vi "Release Buffer.vi"(8 "error in (no error)":errorcluster, 11 "buffer":refnum<data-value>) -> (0 "error out":errorcluster)   [LabVIEW 2017, in "Waveforms (N Ch).lvclass"]
doc: "Releases a reference to a buffer of continuous waveforms. Use this VI to clear all data from the buffer and destroy the buffer reference."
uses:
  <vilib>/addons/_NISVFA/_Shared subVIs/Data Objects/Waveforms (DBL)/Waveforms (N Ch).lvclass
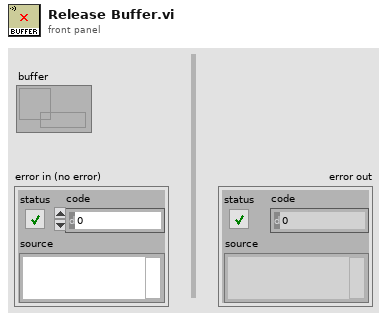
[diagram p1: front panel]
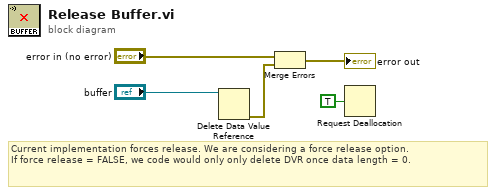
[diagram p0: block diagram]
diagram:
  # "Current implementation forces release. We are considering a force release option. \nIf force release = FALSE, we code would only only delete DVR once data length = 0."
  n1 = Delete Data Value Reference(data value reference="buffer") -> (error out=w2:errorcluster)  [unwired: 1 in, 1 out]
  n2 = Merge Errors("error in (no error)", w2) -> (→"error out":errorcluster)
  n3 = Request Deallocation(TRUE ("flag")) -> ()
